vi "IniNASinfo.vi"(8 "error in":errorcluster, 10 "Report_Time section":string="NAS", 11 "INI file path":path=path "D:/ZDX201 塗膠螺絲鎖固自動化_鴻海/ZDX201_LabView/iniData/NAS_IniData.ini") -> (0 "error out":errorcluster, 1 "NAS_dest":string, 2 "ConnToNAS":string, 3 "Moving_Interval":u32, 4 "DEST":path, 5 "value":bool, 6 "SORC":path)   [LabVIEW 2019]
uses:
  <vilib>/Utility/config.llb/Read Key (String).vi
  <vilib>/Utility/config.llb/Read Key (Path).vi
  <vilib>/Utility/config.llb/Read Key (U32).vi
  <vilib>/Utility/config.llb/Read Key (Boolean).vi
  <vilib>/Utility/config.llb/NI_LVConfig.lvlib
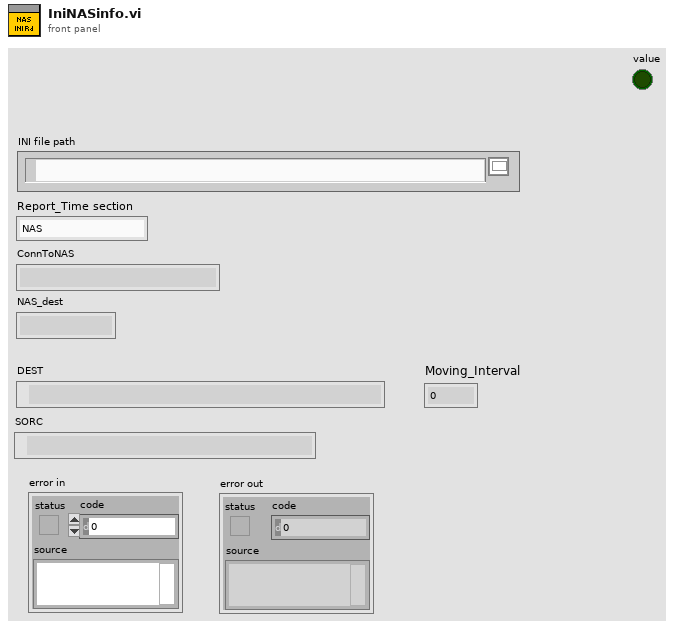
[diagram p1: front panel]
types:
  T1 = typedef "NI_LVConfig.lvlib/Config Data RefNum.ctl" = refnum<k1>
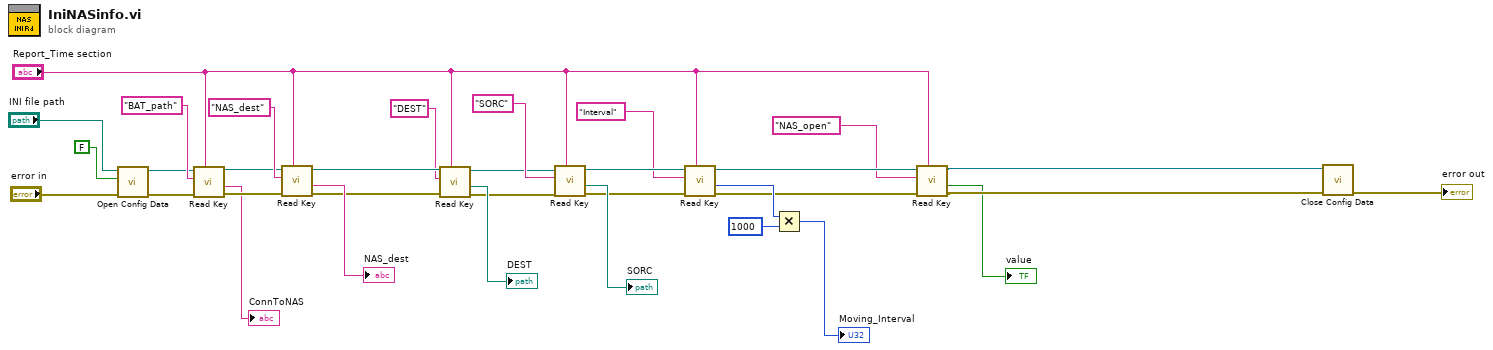
[diagram p0: block diagram]
diagram:
  n1 = call <vilib>:"Open Config Data.vi"("error in (no error)"="error in", "create file if necessary (T)"=FALSE ("create file if necessary? (T)"), "configuration file path"="INI file path") -> ("error out"=w31:errorcluster, "refnum"=w29:T1)  [unwired: 6 in, 1 out]
  n2 = call-poly <vilib>:"Read Key.vi"("section"="Report_Time section", "error in (no error)"=w31, "key"="BAT_path", "refnum"=w29) -> ("error out"=w24:errorcluster, "value"=→"ConnToNAS":string, "refnum out"=w25:T1)  [unwired: 2 in, 3 out]
  n3 = call-poly <vilib>:"Read Key.vi"("section"="Report_Time section", "error in (no error)"=w24, "key"="NAS_dest", "refnum"=w25) -> ("error out"=w21:errorcluster, "value"=→"NAS_dest":string, "refnum out"=w20:T1)  [unwired: 2 in, 3 out]
  n4 = call-poly <vilib>:"Read Key.vi"("section"="Report_Time section", "error in (no error)"=w21, "key"="DEST", "refnum"=w20) -> ("error out"=w15:errorcluster, "value"=→"DEST":path, "refnum out"=w16:T1)  [unwired: 1 in, 4 out]
  n5 = call-poly <vilib>:"Read Key.vi"("section"="Report_Time section", "error in (no error)"=w15, "key"="SORC", "refnum"=w16) -> ("error out"=w12:errorcluster, "value"=→"SORC":path, "refnum out"=w13:T1)  [unwired: 1 in, 4 out]
  n6 = call-poly <vilib>:"Read Key.vi"("section"="Report_Time section", "error in (no error)"=w12, "key"="Interval", "refnum"=w13) -> ("error out"=w6:errorcluster, "value"=w10:u32, "refnum out"=w7:T1)  [unwired: 1 in, 4 out]
  n7 = Multiply(x=w10, y=u32 1000) -> (x*y=→"Moving_Interval":u32)
  n8 = call-poly <vilib>:"Read Key.vi"("section"="Report_Time section", "error in (no error)"=w6, "key"="NAS_open", "refnum"=w7) -> ("error out"=w2:errorcluster, "value"=→"value":bool, "refnum out"=w3:T1)  [unwired: 1 in, 4 out]
  n9 = call <vilib>:"Close Config Data.vi"("error in (no error)"=w2, "refnum"=w3) -> ("error out"=→"error out":errorcluster)  [unwired: 1 in, 8 out]
